vi "Calculate FS.vi"(7 "error in (no error)":errorcluster, 9 "Sensor CoreData":T2[](array[typedef]), 10 "Calibration Points":T1[](array[typedef])) -> (0 "error out":errorcluster, 3 "FS Sensor Cluster":cluster{"SensorID":i32, "FS":dbl}[](array[cluster]))   [LabVIEW 2026, in "Analysis.lvlib"]
uses:
  Analysis.lvlib
  controls/Messaging Payloads/Sensor CoreData Cluster.ctl
  controls/UI/Units Enum.ctl
  controls/UI/Signal Enum.ctl
  controls/Messaging Payloads/Calibration Point Table Insert.ctl
  Settings/Settings.lvlib
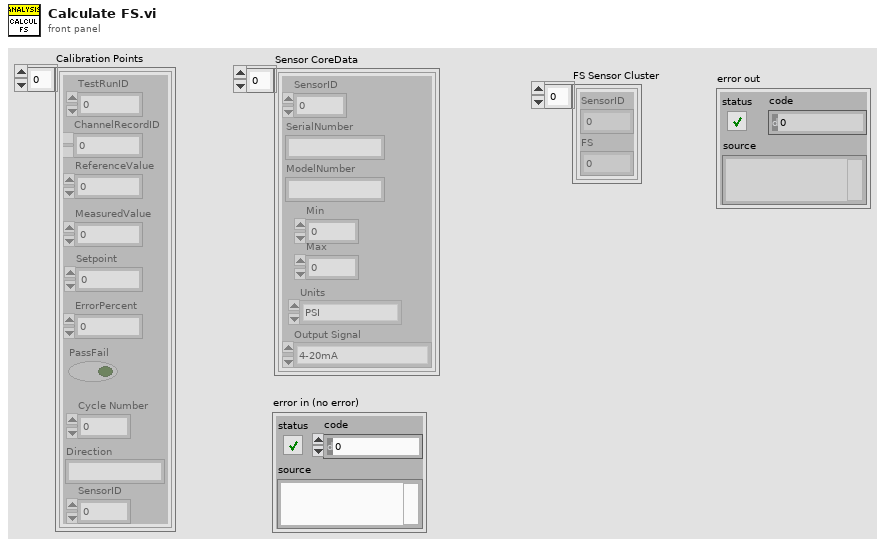
[diagram p1: front panel]
types:
  T1 = typedef "Calibration Point Table Insert.ctl" = cluster{"TestRunID":i32, "ChannelRecordID":i32, "Setpoint":dbl, "MeasuredValue":dbl, "ErrorPercent":dbl, "PassFail":bool, "ReferenceValue":dbl, "Cycle Number":i32, "Direction":string, "SensorID":i32}
  T2 = typedef "Settings.lvlib/Sensor CoreData Cluster.ctl" = cluster{"SensorID":i32, "SerialNumber":string, "ModelNumber":string, "Min":dbl, "Max":dbl, "Units":T3, "Output Signal":T4}
  T3 = typedef "Units Enum.ctl" = enum16{"PSI", "Deg C", "kPa", "GPM"}
  T4 = typedef "Signal Enum.ctl" = enum16{"4-20mA", "0-10V", "Thermocouple Type K"}
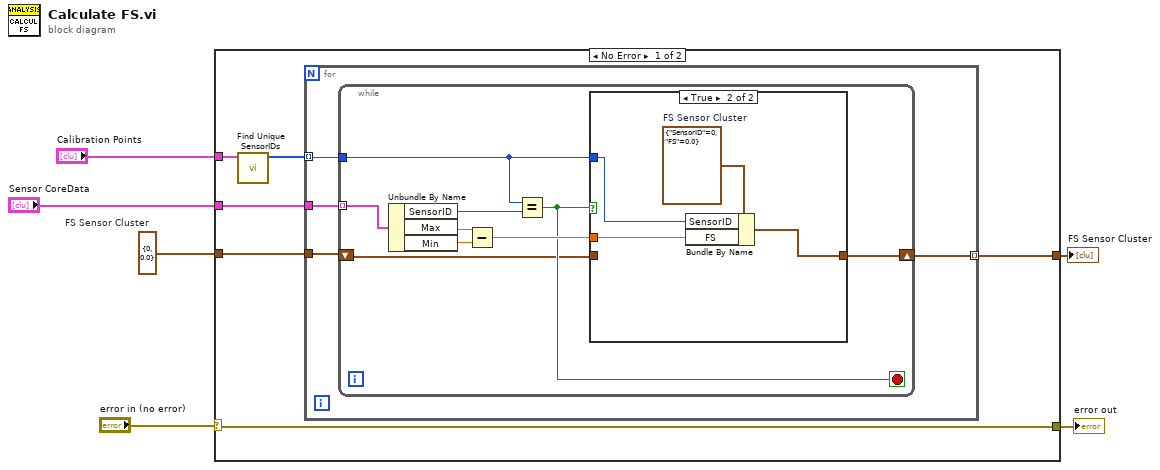
[diagram p0: block diagram]
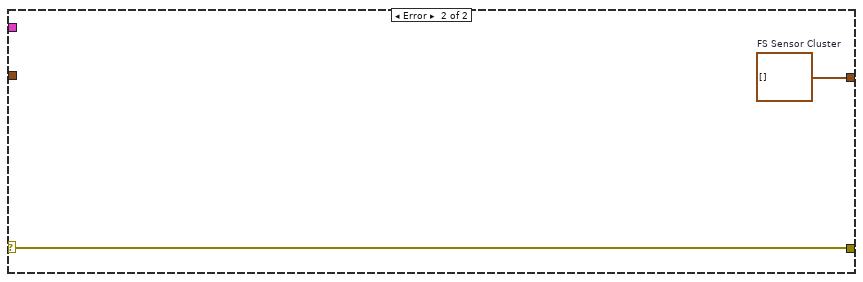
[diagram p3: hidden frame]
diagram:
  w3 = cluster{"SensorID":i32, "FS":dbl} {"SensorID"=0, "FS"=0.0}  # FS Sensor Cluster
  n1 = case shown="No Error" "error in (no error)" {
    selector: "error in (no error)" -> [w7 w32]
    tunnel: "Calibration Points" -> [w12 _]
    tunnel: "Sensor CoreData" -> [w10 _]
    tunnel: [w9 w31] -> w4
    tunnel: w3 -> [w8 _]
    tunnel: [w7 w32] -> w1
    frame No Error {
      n2 = call "Find Unique SensorIDs.vi"("Calibration Points in"=w12) -> ("SensorIDs"=w11:i32[])  [unwired: 9 in, 1 out]
      n3 = for {
        tunnel: [w16] -> w9 mode=indexing
        tunnel: w11 -> [w14] mode=indexing
        tunnel: w10 -> [w15]
        tunnel: w8 -> [w13]
        n4 = while {
          tunnel: w15 -> [w22] mode=indexing
          tunnel: w14 -> [w17]
          shift-right: [w25] -> w16
          shift-left: w13 -> [w18]
          stop <- w19 stop-if-true
          n5 = Unbundle By Name(w22) -> ("SensorID"=w21:i32, "Max"=w23:dbl, "Min"=w24:dbl)
          n6 = Subtract(x=w23, y=w24) -> (x-y=w20:dbl)
          n7 = Equal?(x=w17, y=w21) -> (x = y?=w19:bool)
          n8 = case shown="True" w19 {
            tunnel: [w26 w29] -> w25
            tunnel: w20 -> [_ w28]
            tunnel: w18 -> [w26 _]
            tunnel: w17 -> [_ w27]
            frame False {
            }
            frame True {
              w30 = cluster{"SensorID":i32, "FS":dbl} {"SensorID"=0, "FS"=0.0}  # FS Sensor Cluster
              n9 = Bundle By Name(cluster=w30, "SensorID"=w27, "FS"=w28) -> (w29:cluster{"SensorID":i32, "FS":dbl})
            }
          }
        }
      }
    }
    frame Error {
      w31 = cluster{"SensorID":i32, "FS":dbl}[] []  # FS Sensor Cluster
    }
  }
  "FS Sensor Cluster" <- w4
  "error out" <- w1
